vi "mks946_zero_pressure_channel.vi"(6 "err_in":errorcluster, 7 "visa_in":refnum<visa-resource-name>="COM3", 10 "channel":i32=1, 11 "address":i32=253) -> (0 "status":bool=TRUE, 2 "message":string, 4 "err_out":errorcluster={"status"=FALSE, "code"=1073676294, "source"="VISA Read in thcd_get_chan.vi"}, 5 "visa_out":refnum<visa-resource-name>="COM3")   [LabVIEW 2019]
panel:
  out "type":string
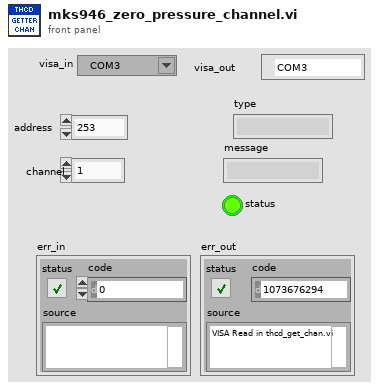
[diagram p1: front panel]
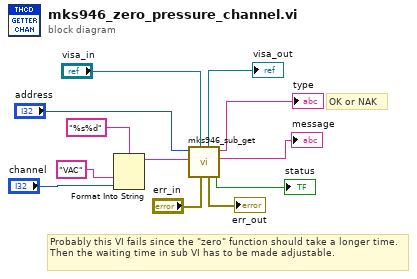
[diagram p0: block diagram]
diagram:
  # "Probably this VI fails since the \"zero\" function should take a longer time.  Then the waiting time in sub VI has to be made adjustable."
  # "OK or NAK"
  n1 = Format Into String(format string="%s%d", "VAC" ("mks946_comm"), "channel") -> (resulting string=w3:string)  [unwired: 2 in, 1 out]
  n2 = call "mks946_sub_get.vi"("error in (no error)"="err_in", "VISA_ref_in"="visa_in", "command"=w3, "address"="address") -> ("status"=→"status":bool, "message"=→"message":string, "response"=→"type":string, "error out"=→"err_out":errorcluster, "VISA_ref_out"=→"visa_out":refnum<visa-resource-name>)  [unwired: 3 in]
